vi "Obtain Recipient.vi"(8 "error in (no error)":errorcluster, 11 "Nested Endpoint in":refnum<class "Nested Endpoint.lvclass">) -> (0 "error out":errorcluster, 2 "Recipient Enqueuer":refnum<class "Message Enqueuer.lvclass">, 3 "Nested Endpoint out":refnum<class "Nested Endpoint.lvclass">)   [LabVIEW 2020, in "Nested Endpoint.lvlib" / "Nested Endpoint.lvclass"]
doc: "This override returns the enqueuer of the enpoint's caller."
uses:
  Nested Endpoint.lvclass
  <vilib>/ActorFramework/Actor/Actor.lvclass
  <vilib>/ActorFramework/Message Enqueuer/Message Enqueuer.lvclass
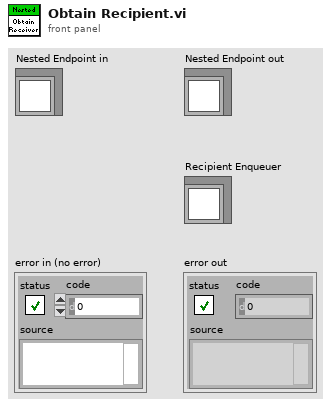
[diagram p1: front panel]
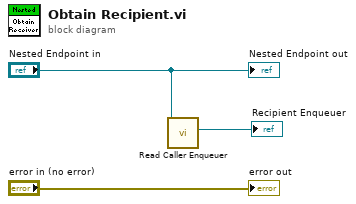
[diagram p0: block diagram]
diagram:
  n1 = call <vilib>:"Read Caller Enqueuer.vi"("Actor"="Nested Endpoint in") -> ("Caller Enqueuer"=→"Recipient Enqueuer":refnum<class "Message Enqueuer.lvclass">)  [unwired: 10 in]
  "error out" <- "error in (no error)"
  "Nested Endpoint out" <- "Nested Endpoint in"
